vi "FinalDemoZoneCounter.vi"() -> ()   [LabVIEW 2016, in "Test.lvrbt"]
uses:
  Test.lvrbt
  <vilib>/NXT/Block Support/NXT_OutputPort.ctl
  <vilib>/NXT/Block Support/NXT_InputPort.ctl
  <vilib>/NXT/Dual Mode Library/Motors/ResetMotor.vi
  <vilib>/NXT/Dual Mode Library/Waits/Wait_Num(msec).vi
  <vilib>/NXT/Dual Mode Library/Display/drawText.vi
  <vilib>/NXT/Dual Mode Library/Sensors/EV3_Color_Reflect.vi
  <vilib>/NXT/Dual Mode Library/Sensors/Touch_Pressed.vi
  <vilib>/NXT/Dual Mode Library/Sensors/EV3_Ultrasonic_CM.vi
  <vilib>/NXT/Dual Mode Library/Display/drawNumber.vi
  <vilib>/NXT/Dual Mode Library/Motors/Rotation.vi
  <vilib>/NXT/NXTIO Xnodes/NXTIONodeSubVIs/NXTMoveMotors.vi
  <vilib>/NXT/NXTIO Xnodes/NXTIONodeSubVIs/NXTMotorRunDistance.vi
  <vilib>/NXT/NXTIO Xnodes/NXTIONodeSubVIs/NXTMotorSteeringOn.vi
  <vilib>/NXT/NXTIO Xnodes/AddressXNode/NXTIOAddress.xnode
  <vilib>/NXT/Subs/LVHSConnector.ctl
  <vilib>/NXT/NXTIO Xnodes/NXTIOXNode/NXTIO.xnode
  <vilib>/NXT/LegoClasses/BrickReference/BrickReference.lvclass
panel:
  out "Combined 2":dbl(graph)
  out "kP 2":sgl(graph)
  out "kI 2":dbl(graph)
  out "kD 2":dbl(graph)
  out "rotation":dbl
  out "Zone Detector":dbl
  out "Box Number":dbl
  out "Power Sum":dbl
  out "Distance":dbl
  out "button":bool
  out "power":dbl
  out "Combined":dbl(graph)
  out "kP":sgl(graph)
  out "kI":dbl(graph)
  out "kD":dbl(graph)
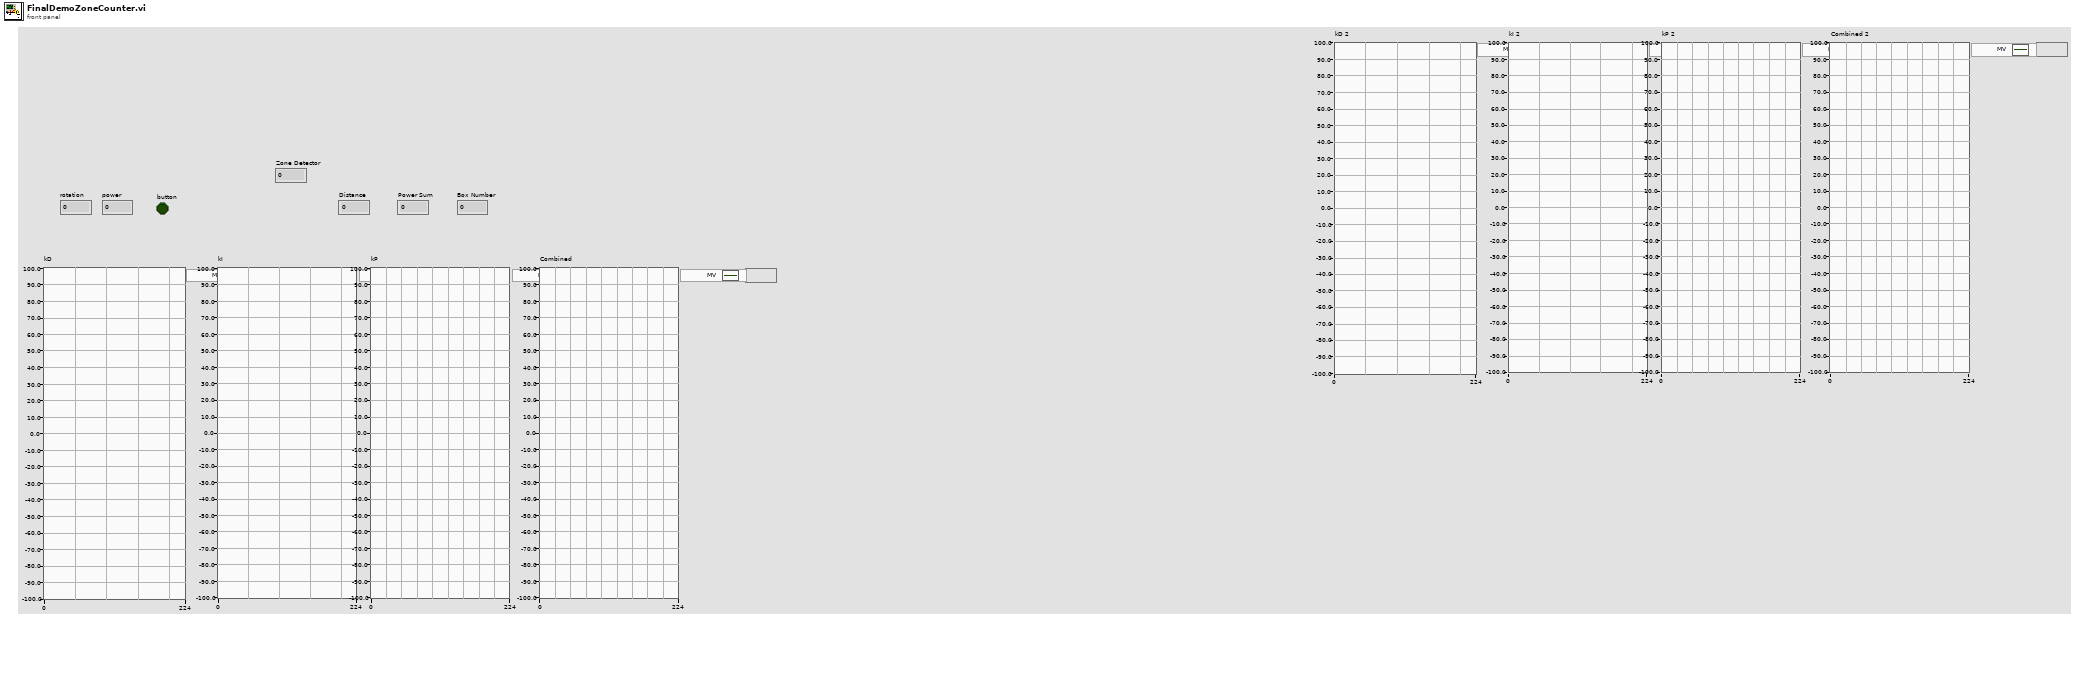
[diagram p1: front panel]
types:
  T1 = typedef "NXT_OutputPort.ctl" = u8
  T2 = typedef "NXT_InputPort.ctl" = u32
  T3 = typedef "LVHSConnector.ctl" = refnum<class "BrickReference.lvclass">
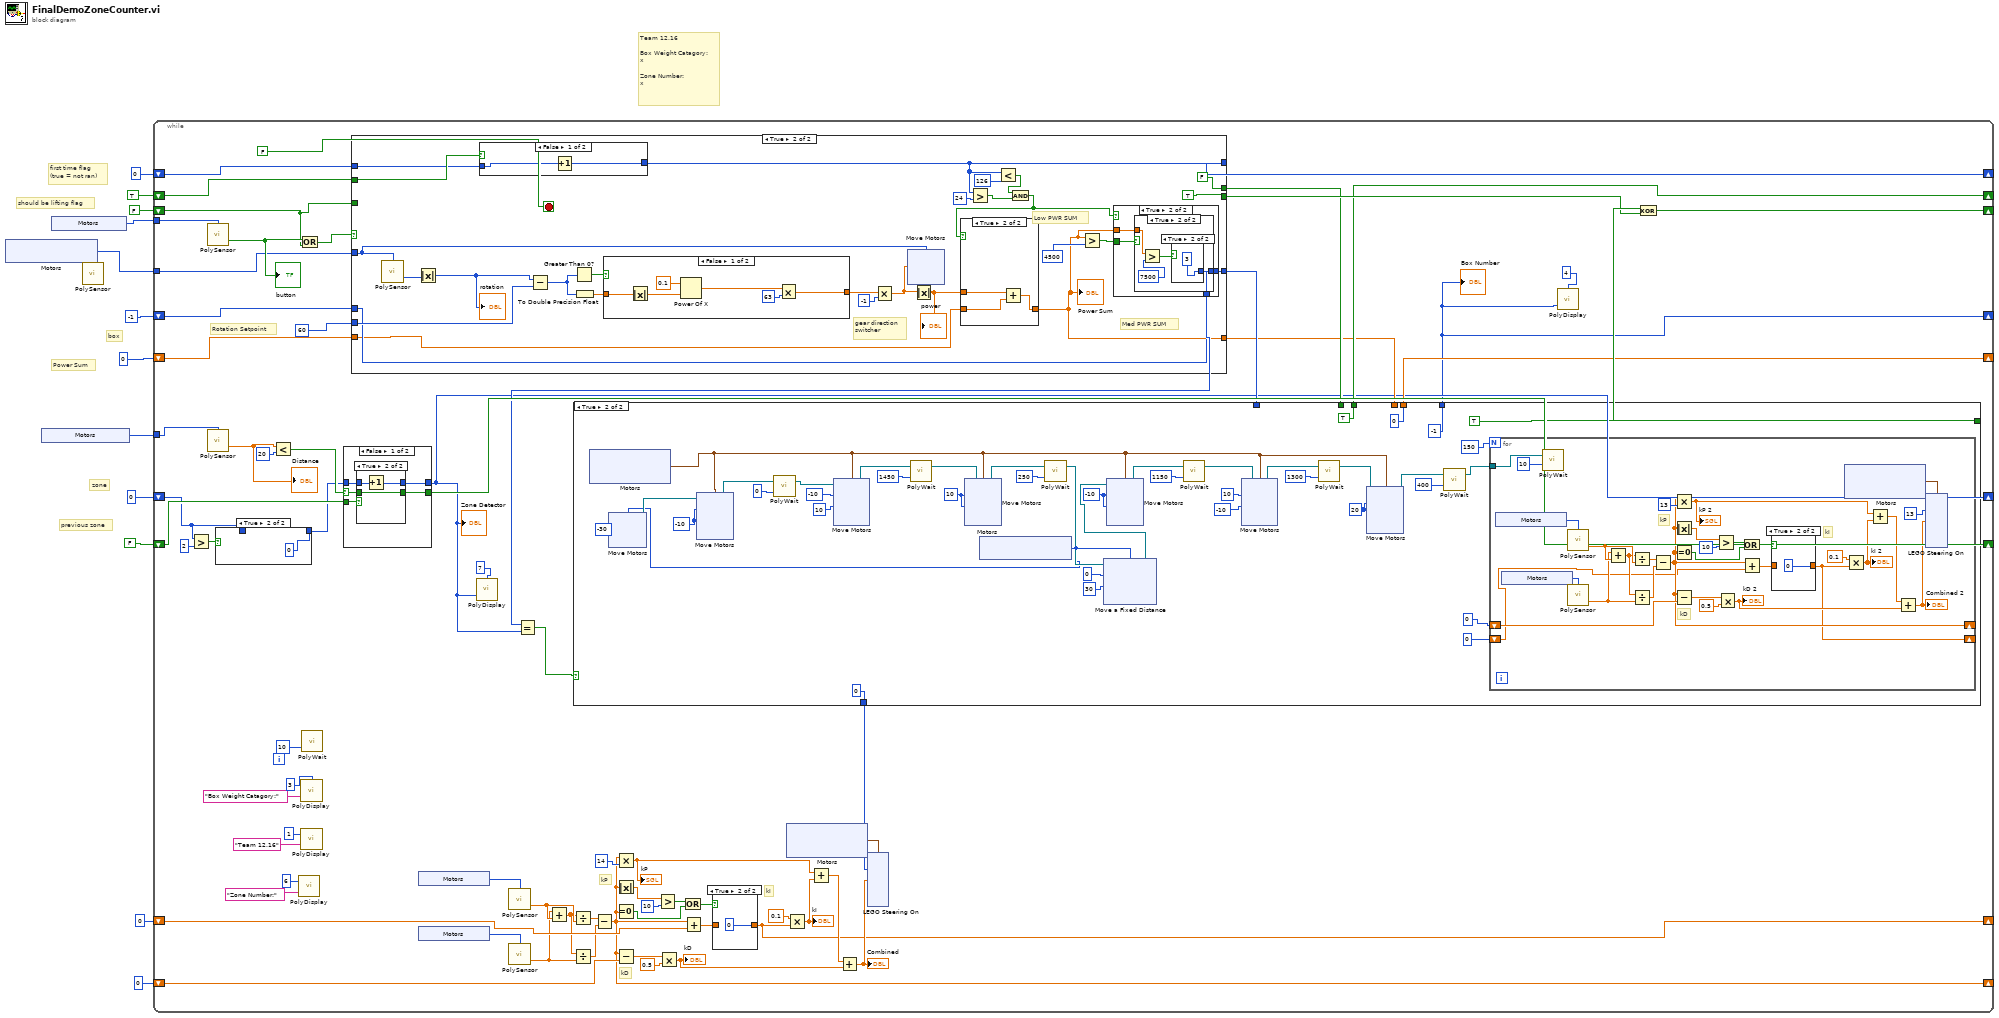
[diagram p0: block diagram]
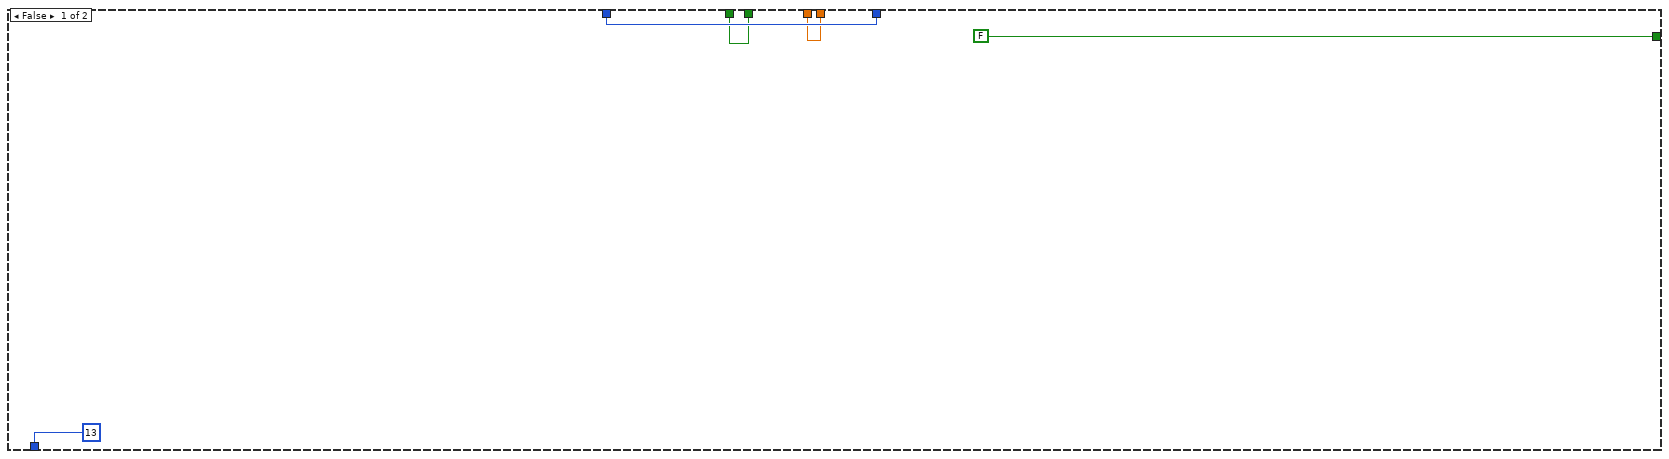
[diagram p5: hidden frame]
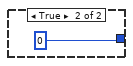
[diagram p8: hidden frame]
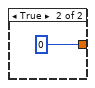
[diagram p10: hidden frame]
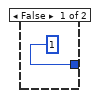
[diagram p12: hidden frame]
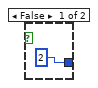
[diagram p13: hidden frame]
diagram:
  # "box"
  # "zone"
  # "previous zone"
  # "Team 12.16\n\nBox Weight Catagory:\nx\n\nZone Number:\nx"
  # "should be lifting flag"
  # "first time flag\n(true = not ran)"
  # "Power Sum"
  n1 = xnode "Motors"() -> ("Motor"=w1:T1)
  n2 = xnode "Motors"() -> ("Sensor"=w9:T2)
  n3 = xnode "Motors"() -> ("Sensor"=w8:T2)
  n4 = call-poly <vilib>:"PolySensor.vi"("Port (All Ports)"=w1) -> ()  [unwired: 3 in, 1 out]
  n5 = while {
    shift-right: [w54] -> _
    shift-left: 0 -> [w81]
    shift-right: [w55] -> _
    shift-left: 0 -> [w80]
    tunnel: w1 -> [w36]
    shift-right: [w52] -> _
    shift-left: FALSE -> [w48]
    tunnel: w9 -> [w45]
    tunnel: w8 -> [w46]
    shift-right: [w13] -> _
    shift-left: -1 -> [w44]
    shift-right: [w18] -> _
    shift-left: TRUE -> [w43]
    shift-right: [w16] -> _
    shift-left: 0 -> [w40]
    shift-right: [w38] -> _
    shift-left: u32 0 ("Time (100 msec)") -> [w39]
    shift-right: [w25] -> _
    shift-left: FALSE -> [w26]
    shift-right: [w14] -> _
    shift-left: 0 -> [w20]
    stop <- FALSE stop-if-true
    # "Rotation Setpoint"
    # "kD"
    # "kI"
    # "kP"
    n6 = Greater?(x=w20, y=2 ("x")) -> (0:w22:bool)
    n7 = call-poly <vilib>:"PolySensor.vi"("Port (Port 1)"=w46) -> ("Yes / No"=w57:bool)  [unwired: 2 in, 1 out]
    "button" <- w57
    n8 = call-poly <vilib>:"PolySensor.vi"("Port (Port 1)"=w45) -> ("Centimeters"=w42:sgl)  [unwired: 2 in, 1 out]
    "Distance" <- w42
    n9 = case shown="True" w22 {
      tunnel: [w83 0] -> w19
      tunnel: w20 -> [w83 _]
      frame False {
      }
      frame True {
      }
    }
    n10 = Less?(x=w42, y=20) -> (x < y?=w27:bool)
    n11 = call-poly <vilib>:"PolyDisplay.vi"("Text"="Zone Number:", "Line"=6 ("number")) -> ()  [unwired: 2 in, 1 out]
    n12 = Or(x=w57, y=w48) -> (x .or. y?=w56:bool)
    n13 = call-poly <vilib>:"PolyDisplay.vi"("Text"="Box Weight Catagory:", "Line"=3 ("number")) -> ()  [unwired: 2 in, 1 out]
    n14 = call-poly <vilib>:"PolyDisplay.vi"("Text"="Team 12.16", "Line"=1 ("number")) -> ()  [unwired: 2 in, 1 out]
    n15 = call-poly <vilib>:"PolyWait.vi"("Time (100 msec)"=u32 10) -> ()  [unwired: 3 in, 1 out]
    n16 = case shown="False" w27 {
      selector: w27 -> [w85 w95]
      tunnel: w26 -> [w89 _]
      tunnel: [w88 w96] -> w14
      tunnel: w19 -> [w87 w96]
      tunnel: [w86 w95] -> w25
      frame False {
        n17 = case shown="True" w89 {
          selector: w89 -> [w90 _]
          tunnel: [w91 w93] -> w88
          tunnel: w87 -> [w91 w94]
          tunnel: [w90 w92] -> w86
          tunnel: w85 -> [_ w92]
          frame False {
          }
          frame True {
            n18 = Increment(x=w94) -> (x+1=w93:i32)
          }
        }
      }
      frame True {
      }
    }
    "Zone Detector" <- w14
    n19 = case shown="True" w56 {
      tunnel: w36 -> [_ w284]
      tunnel: 60 -> [_ w283]
      tunnel: [w257 TRUE] -> w49
      tunnel: w48 -> [w257 _]
      tunnel: [w256 w279] -> w23
      tunnel: w44 -> [w256 w278]
      tunnel: [w255 FALSE] -> w17
      tunnel: w43 -> [w255 w271]
      tunnel: w40 -> [w254 w273]
      tunnel: [w254 w272] -> w15
      tunnel: w39 -> [w253 w270]
      tunnel: [w253 w269] -> w38
      frame False {
      }
      frame True {
        # "gear direction\nswitcher"
        # "Med PWR SUM"
        # "Low PWR SUM"
        n20 = call-poly <vilib>:"PolySensor.vi"("Port (Port A)"=w284) -> ("Angle of Rotation"=w265:i32)  [unwired: 2 in, 1 out]
        n21 = Absolute Value(x=w265) -> (abs(x)=w264:i32)
        "rotation" <- w264
        n22 = case shown="False" w271 {
          tunnel: [w285 u32 0 ("Time (100 msec)")] -> w269
          tunnel: w270 -> [w286 _]
          frame False {
            n23 = Increment(x=w286) -> (x+1=w285:u32)
          }
          frame True {
          }
        }
        n24 = Subtract(x=w264, y=w283) -> (x-y=w277:i32)
        n25 = Greater Than 0?(x=w277) -> (x > 0?=w276:bool)
        n26 = To Double Precision Float(number=w277) -> (double precision float=w275:dbl)
        n27 = case shown="False" w276 {
          tunnel: [w294 0] -> w261
          tunnel: w275 -> [w293 _]
          frame False {
            n28 = Absolute Value(x=w293) -> (abs(x)=w292:dbl)
            n29 = Power Of X(1:w292, 2:0.1) -> (0:w295:dbl)
            n30 = Multiply(x=w295, y=63) -> (x*y=w294:dbl)
          }
          frame True {
          }
        }
        n31 = Multiply(x=w261, y=-1) -> (x*y=w260:dbl)
        n32 = xnode "Move Motors"("Power/Speed 1"=w260, "Motors"=w284) -> ()  [unwired: 1 in, 1 out]
        n33 = Absolute Value(x=w260) -> (abs(x)=w263:dbl)
        "power" <- w263
        n34 = Greater?(x=w269, y=24) -> (0:w266:bool)
        n35 = Less?(x=w269, y=126) -> (x < y?=w267:bool)
        n36 = And(x=w267, y=w266) -> (x .and. y?=w258:bool)
        n37 = case shown="True" w258 {
          tunnel: w263 -> [_ w291]
          tunnel: [w288 w290] -> w272
          tunnel: w273 -> [w288 w289]
          frame False {
          }
          frame True {
            n38 = Add(x=w291, y=w289) -> (x+y=w290:dbl)
          }
        }
        "Power Sum" <- w272
        n39 = Greater?(x=w272, y=4500) -> (0:w281:bool)
        n40 = case shown="True" w258 {
          tunnel: w281 -> [_ w309]
          tunnel: [w306 w308] -> w279
          tunnel: w272 -> [_ w307]
          tunnel: w278 -> [w306 _]
          frame False {
          }
          frame True {
            n41 = case shown="True" w309 {
              tunnel: [1 w311] -> w308
              tunnel: w307 -> [_ w313]
              frame False {
              }
              frame True {
                n42 = Greater?(x=w313, y=7500) -> (0:w314:bool)
                n43 = case shown="True" w314 {
                  tunnel: [2 3] -> w311
                  frame False {
                  }
                  frame True {
                  }
                }
              }
            }
          }
        }
      }
    }
    n44 = xnode "Motors"() -> ("Sensor"=w50:T2)
    n45 = xnode "Motors"() -> ("Sensor"=w79:T2)
    n46 = call-poly <vilib>:"PolyDisplay.vi"("number"=w14, "Line"=7 ("number")) -> ()  [unwired: 2 in, 1 out]
    n47 = call-poly <vilib>:"PolySensor.vi"("Port (Port 1)"=w50) -> ("Scaled Value"=w78:sgl)  [unwired: 2 in, 1 out]
    n48 = call-poly <vilib>:"PolySensor.vi"("Port (Port 1)"=w79) -> ("Scaled Value"=w77:sgl)  [unwired: 2 in, 1 out]
    n49 = Equal?(x=w23, y=w14) -> (x = y?=w41:bool)
    n50 = Add(x=w77, y=w78) -> (x+y=w76:sgl)
    n51 = Divide(x=w76, y=w78) -> (x/y=w75:sgl)
    n52 = Divide(x=w76, y=w77) -> (x/y=w73:sgl)
    n53 = case shown="True" w41 {
      tunnel: [FALSE TRUE] -> w51
      tunnel: [13 0] -> w35
      tunnel: [w99 -1] -> w13
      tunnel: w23 -> [w99 _]
      tunnel: [w98 TRUE] -> w18
      tunnel: w17 -> [w98 _]
      tunnel: [w97 0] -> w16
      tunnel: w15 -> [w97 _]
      frame False {
      }
      frame True {
        w102 = i8 20 ("Power/Speed 1")
        w115 = i8 -10 ("Power/Speed 2")
        w129 = i8 -10 ("Power/Speed 2")
        w131 = i8 10 ("Power/Speed 2")
        n54 = xnode "Motors"() -> ("Motor"=w103:cluster{"Port":T1, "Port":T1})
        n55 = xnode "Motors"() -> ("Motor"=w112:T1)
        n56 = xnode "Move Motors"("Power/Speed 1"=i8 -30 ("Power/Speed 2"), "Motors"=w112) -> ("NXT/EV3"=w113:T3)  [unwired: 1 in]
        n57 = xnode "Move Motors"("Power/Speed 2"=w115, "Power/Speed 1"=w115, "Motors"=w103, "NXT/EV3"=w113) -> ("NXT/EV3"=w118:T3)
        n58 = call-poly <vilib>:"PolyWait.vi"("Time (100 msec)"=u32 0, "NXT/EV3"=w118) -> ("NXT/EV3"=w116:T3)  [unwired: 2 in]
        n59 = xnode "Move Motors"("Power/Speed 2"=i8 10, "Power/Speed 1"=i8 -10, "Motors"=w103, "NXT/EV3"=w116) -> ("NXT/EV3"=w138:T3)
        n60 = call-poly <vilib>:"PolyWait.vi"("Time (100 msec)"=u32 1450, "NXT/EV3"=w138) -> ("NXT/EV3"=w134:T3)  [unwired: 2 in]
        n61 = xnode "Move Motors"("Power/Speed 2"=w131, "Power/Speed 1"=w131, "Motors"=w103, "NXT/EV3"=w134) -> ("NXT/EV3"=w136:T3)
        n62 = call-poly <vilib>:"PolyWait.vi"("Time (100 msec)"=u32 250, "NXT/EV3"=w136) -> ("NXT/EV3"=w130:T3)  [unwired: 2 in]
        n63 = xnode "Move a Fixed Distance"("Speed 1"=i8 30 ("Power/Speed 2"), "Distance 1"=i8 0 ("Power/Speed 2"), "Motors"=w112, "NXT/EV3"=w130) -> ("NXT/EV3"=w114:T3)
        n64 = xnode "Move Motors"("Power/Speed 2"=w129, "Power/Speed 1"=w129, "Motors"=w103, "NXT/EV3"=w114) -> ("NXT/EV3"=w127:T3)
        n65 = call-poly <vilib>:"PolyWait.vi"("Time (100 msec)"=u32 1150, "NXT/EV3"=w127) -> ("NXT/EV3"=w122:T3)  [unwired: 2 in]
        n66 = xnode "Move Motors"("Power/Speed 2"=i8 -10, "Power/Speed 1"=i8 10, "Motors"=w103, "NXT/EV3"=w122) -> ("NXT/EV3"=w125:T3)
        n67 = call-poly <vilib>:"PolyWait.vi"("Time (100 msec)"=u32 1300, "NXT/EV3"=w125) -> ("NXT/EV3"=w106:T3)  [unwired: 2 in]
        n68 = xnode "Move Motors"("Power/Speed 2"=w102, "Power/Speed 1"=w102, "Motors"=w103, "NXT/EV3"=w106) -> ("NXT/EV3"=w105:T3)
        n69 = call-poly <vilib>:"PolyWait.vi"("Time (100 msec)"=u32 400, "NXT/EV3"=w105) -> ("NXT/EV3"=w104:T3)  [unwired: 2 in]
        n70 = for {
          N: u32 150 ("Time (100 msec)") -> [_]
          shift-right: [w156] -> _
          shift-left: u32 0 ("Time (100 msec)") -> [w157]
          shift-right: [w154] -> _
          shift-left: u32 0 ("Time (100 msec)") -> [w155]
          tunnel: w104 -> [w152]
          # "kD"
          # "kI"
          # "kP"
          n71 = xnode "Motors"() -> ("Sensor"=w159:T2)
          n72 = xnode "Motors"() -> ("Sensor"=w180:T2)
          n73 = call-poly <vilib>:"PolyWait.vi"("Time (100 msec)"=u32 10, "NXT/EV3"=w152) -> ()  [unwired: 2 in, 1 out]
          n74 = call-poly <vilib>:"PolySensor.vi"("Port (Port 1)"=w159) -> ("Scaled Value"=w179:sgl)  [unwired: 2 in, 1 out]
          n75 = call-poly <vilib>:"PolySensor.vi"("Port (Port 1)"=w180) -> ("Scaled Value"=w178:sgl)  [unwired: 2 in, 1 out]
          n76 = Add(x=w178, y=w179) -> (x+y=w177:sgl)
          n77 = Divide(x=w177, y=w179) -> (x/y=w176:sgl)
          n78 = Divide(x=w177, y=w178) -> (x/y=w174:sgl)
          n79 = Subtract(x=w176, y=w174) -> (x-y=w156:sgl)
          n80 = Multiply(x=w156, y=13) -> (x*y=w161:sgl)
          "kP 2" <- w161
          n81 = Absolute Value(x=w156) -> (abs(x)=w169:sgl)
          n82 = Equal To 0?(x=w156) -> (x = 0?=w171:bool)
          n83 = Subtract(x=w156, y=w157) -> (x-y=w166:sgl)
          n84 = Greater?(x=w169, y=10) -> (0:w168:bool)
          n85 = Multiply(x=w166, y=0.5) -> (x*y=w163:dbl)
          "kD 2" <- w163
          n86 = Or(x=w168, y=w171) -> (x .or. y?=w170:bool)
          n87 = Add(x=w156, y=w155) -> (x+y=w173:sgl)
          n88 = case shown="True" w170 {
            tunnel: w173 -> [w181 _]
            tunnel: [w181 0] -> w154
            frame False {
            }
            frame True {
            }
          }
          n89 = xnode "Motors"() -> ("Motor"=w158:cluster{"Port":T1, "Port":T1})
          n90 = Multiply(x=0.1, y=w154) -> (x*y=w162:dbl)
          "kI 2" <- w162
          n91 = Add(x=w161, y=w162) -> (x+y=w164:dbl)
          n92 = Add(x=w164, y=w163) -> (x+y=w160:dbl)
          "Combined 2" <- w160
          n93 = xnode "LEGO Steering On"("Steering 1"=w160, "Power 1"=u32 13 ("Time (100 msec)"), "Motors"=w158) -> ()  [unwired: 1 in, 1 out]
        }
      }
    }
    "Box Number" <- w13
    n94 = Subtract(x=w75, y=w73) -> (x-y=w55:sgl)
    n95 = Multiply(x=w55, y=14) -> (x*y=w60:sgl)
    "kP" <- w60
    n96 = Absolute Value(x=w55) -> (abs(x)=w68:sgl)
    n97 = Equal To 0?(x=w55) -> (x = 0?=w70:bool)
    n98 = Subtract(x=w55, y=w80) -> (x-y=w65:sgl)
    n99 = Greater?(x=w68, y=10) -> (0:w67:bool)
    n100 = Multiply(x=w65, y=0.5) -> (x*y=w62:dbl)
    "kD" <- w62
    n101 = Or(x=w67, y=w70) -> (x .or. y?=w69:bool)
    n102 = Add(x=w55, y=w81) -> (x+y=w72:sgl)
    n103 = case shown="True" w69 {
      tunnel: w72 -> [w317 _]
      tunnel: [w317 0] -> w54
      frame False {
      }
      frame True {
      }
    }
    n104 = xnode "Motors"() -> ("Motor"=w24:cluster{"Port":T1, "Port":T1})
    n105 = Multiply(x=0.1, y=w54) -> (x*y=w61:dbl)
    "kI" <- w61
    n106 = Add(x=w60, y=w61) -> (x+y=w63:dbl)
    n107 = Add(x=w63, y=w62) -> (x+y=w59:dbl)
    "Combined" <- w59
    n108 = xnode "LEGO Steering On"("Steering 1"=w59, "Power 1"=w35, "Motors"=w24) -> ()  [unwired: 1 in, 1 out]
    n109 = call-poly <vilib>:"PolyDisplay.vi"("number"=w13, "Line"=4 ("number")) -> ()  [unwired: 2 in, 1 out]
    n110 = Exclusive Or(1:w49, 2:w51) -> (0:w52:bool)
  }
